vi "AcPwrClass.vi"(7 "btnSet":bool caption="Set? (F)", 11 "Class In":refnum<class "AcPwrBase.lvclass">) -> (3 "Class Out":refnum<class "AcPwrBase.lvclass">)   [LabVIEW 2018, in "AcPwrPlugins.lvlib"]
uses:
  AcPwrPlugins.lvlib
  AcPwrBaseClass/AcPwrBase.lvclass
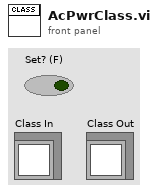
[diagram p1: front panel]
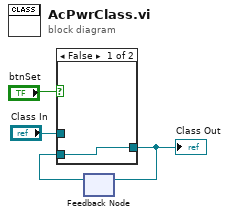
[diagram p0: block diagram]
diagram:
  n1 = feedback #1() -> (w1:refnum<class "AcPwrBase.lvclass">)  [unwired: 1 in]
  n2 = case shown="False" "btnSet" {
    tunnel: [w5 w6] -> w2
    tunnel: "Class In" -> [_ w6]
    tunnel: w1 -> [w5 _]
    frame False {
    }
    frame True {
    }
  }
  "Class Out" <- w2
  n3 = feedback-in #1(w2) -> ()
